vi "InitializeMotor.vi"(8 "error in":errorcluster) -> (0 "error out":errorcluster, 3 "Motor Ref":T1)   [LabVIEW 2016]
uses:
  <vilib>/myRIO/Instrument Drivers/Onboard IO/PWM/typedefs/PWM Configuration.ctl
  <vilib>/myRIO/Instrument Drivers/Onboard IO/PWM/PWM.lvlib
  <vilib>/myRIO/Common/Instrument Driver Framework/myRIO v1.0/PWM/typedefs/PWM Channels Enum.ctl
  <vilib>/myRIO/Common/Instrument Driver Framework/Utilities/typedefs/Generic FPGA Reference.ctl
  <vilib>/myRIO/Common/Instrument Driver Framework/Utilities/typedefs/myRIO v1.0 Reference.ctl
  <vilib>/myRIO/Common/Instrument Driver Framework/Utilities/typedefs/Hardware Version Enum.ctl
  <vilib>/myRIO/Common/Instrument Driver Framework/Utilities/typedefs/myRIO Generic Hardware Reference.ctl
  <vilib>/myRIO/Instrument Drivers/Onboard IO/PWM/typedefs/PWM Reference.ctl
  <vilib>/myRIO/Instrument Drivers/Onboard IO/PWM/vis/myRIO PWM Open.xnode
  <vilib>/myRIO/Common/Instrument Driver Framework/myRIO v1.0/PWM/vis/myRIO v1.1 Open PWM.vi
  <vilib>/userdefined/High Color/nirio_resource_hc.ctl
  <vilib>/myRIO/Common/Instrument Driver Framework/myRIO v1.0/DIO/typedefs/DIO Channels Enum.ctl
  <vilib>/myRIO/Common/Instrument Driver Framework/myRIO v1.0/DIO/typedefs/DIO Channels List.ctl
  <vilib>/myRIO/Instrument Drivers/Onboard IO/DIO/typedefs/DIO Reference.ctl
  <vilib>/myRIO/Instrument Drivers/Onboard IO/DIO/DIO.lvlib
  <vilib>/myRIO/Instrument Drivers/Onboard IO/DIO/vis/myRIO DIO Open.xnode
  <vilib>/myRIO/Common/Instrument Driver Framework/myRIO v1.0/DIO/vis/myRIO v1.1 Open DIO.vi
  <vilib>/myRIO/Common/Instrument Driver Framework/myRIO v1.0/Encoder/typedefs/Encoder Channels Enum.ctl
  <vilib>/myRIO/Instrument Drivers/Onboard IO/Encoder/typedefs/Encoder Reference.ctl
  <vilib>/myRIO/Instrument Drivers/Onboard IO/Encoder/Encoder.lvlib
  <vilib>/myRIO/Common/Instrument Driver Framework/myRIO v1.0/Encoder/typedefs/Encoder Signal Mode.ctl
  <vilib>/myRIO/Instrument Drivers/Onboard IO/Encoder/vis/myRIO Encoder Open.xnode
  <vilib>/myRIO/Common/Instrument Driver Framework/myRIO v1.0/Encoder/vis/myRIO v1.1 Open Encoder.vi
  <vilib>/myRIO/Common/Instrument Driver Framework/myRIO v1.0/Encoder/vis/myRIO v1.0 Configure Encoder.vi
  <vilib>/myRIO/Common/Instrument Driver Framework/myRIO v1.0/Encoder/typedefs/Encoder Configuration v1.0.ctl
  MotorObject.ctl
panel:
  in  "Motor Object":T1
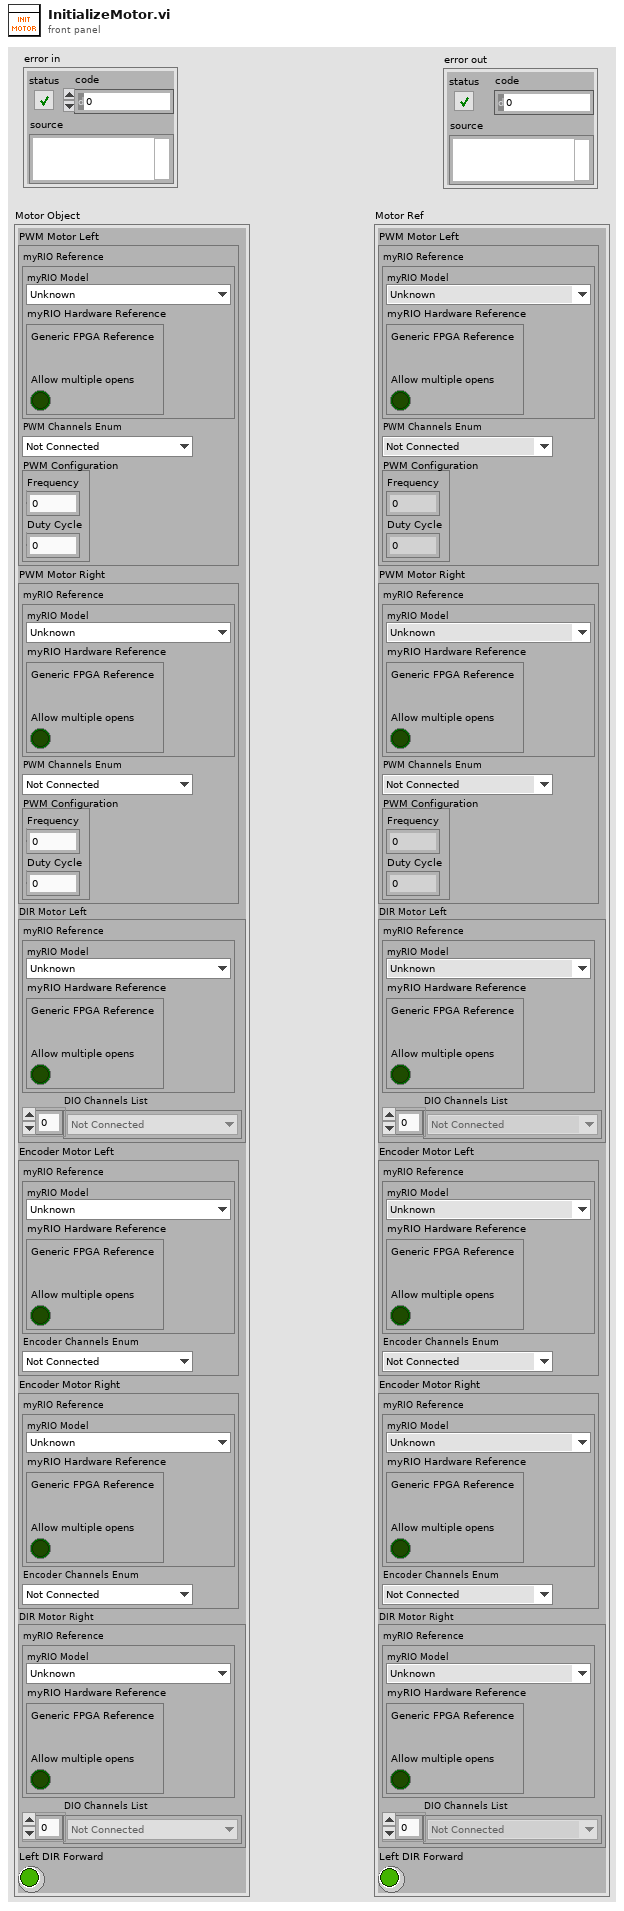
[diagram p1: front panel]
types:
  T1 = typedef "MotorObject.ctl" = cluster{"PWM Motor Left":T2, "PWM Motor Right":T2, "DIR Motor Left":T9, "Encoder Motor Left":T12, "Encoder Motor Right":T12, "DIR Motor Right":T9, "Left DIR Forward":bool}
  T2 = typedef "PWM.lvlib/PWM Reference.ctl" = cluster{"myRIO Reference":T3, "PWM Channels Enum":T7, "PWM Configuration":T8}
  T3 = typedef "myRIO Generic Hardware Reference.ctl" = cluster{"myRIO Model":T4, "myRIO Hardware Reference":T5}
  T4 = typedef "Hardware Version Enum.ctl" = enum16{"Unknown", "myRIO-1900", "myRIO-1950", "roboRIO", "NI ELVIS RIO CM"}
  T5 = typedef "myRIO v1.0 Reference.ctl" = cluster{"Generic FPGA Reference":T6, "Allow multiple opens":bool}
  T6 = typedef "Generic FPGA Reference.ctl" = refnum<k20>
  T7 = typedef "PWM Channels Enum.ctl" = enum16{"Not Connected", "C/PWM0", "C/PWM1", "A/PWM0", "A/PWM1", "A/PWM2", "B/PWM0", "B/PWM1", "B/PWM2", "PWM/PWM0", "PWM/PWM1", "PWM/PWM2", "PWM/PWM3", "PWM/PWM4", "PWM/PWM5", "PWM/PWM6", "PWM/PWM7", "PWM/PWM8", "PWM/PWM9"}
  T8 = typedef "PWM.lvlib/PWM Configuration.ctl" = cluster{"Frequency":dbl, "Duty Cycle":dbl}
  T9 = typedef "DIO.lvlib/DIO Reference.ctl" = cluster{"myRIO Reference":T3, "DIO Channels List":T10}
  T10 = typedef "DIO Channels List.ctl" = T11[]
  T11 = typedef "DIO Channels Enum.ctl" = enum16{"Not Connected", "C/DIO0", "C/DIO1", "C/DIO2", "C/DIO3", "C/DIO4", "C/DIO5", "C/DIO6", "C/DIO7", "A/DIO0", "A/DIO1", "A/DIO2", "A/DIO3", "A/DIO4", "A/DIO5", "A/DIO6", "A/DIO7", "A/DIO8", "A/DIO9", "A/DIO10", "A/DIO11", "A/DIO12", "A/DIO13", "A/DIO14", "A/DIO15", "B/DIO0", "B/DIO1", "B/DIO2", "B/DIO3", "B/DIO4", "B/DIO5", "B/DIO6", "B/DIO7", "B/DIO8", "B/DIO9", "B/DIO10", "B/DIO11", "B/DIO12", "B/DIO13", "B/DIO14", "B/DIO15", "LED0", "LED1", "LED2", "LED3", "Button0", "DIO/DIO0", "DIO/DIO1", "DIO/DIO2", "DIO/DIO3", "DIO/DIO4", "DIO/DIO5", "DIO/DIO6", "DIO/DIO7", "DIO/DIO8", "DIO/DIO9", "SPI/CS0", "SPI/CS1", "SPI/CS2", "SPI/CS3", "LED RADIO (Green)", "LED RADIO (Red)", "LED COMM (Green)", "LED COMM (Red)", "LED MODE (Green)", "LED MODE (Red)"}
  T12 = typedef "Encoder.lvlib/Encoder Reference.ctl" = cluster{"myRIO Reference":T3, "Encoder Channels Enum":T13}
  T13 = typedef "Encoder Channels Enum.ctl" = enum16{"Not Connected", "C/ENC0", "C/ENC1", "A/ENC", "B/ENC", "DIO/ENC0", "DIO/ENC1", "DIO/ENC2", "DIO/ENC3", "DIO/ENC4"}
  T14 = typedef "nirio_resource_hc.ctl" = tag
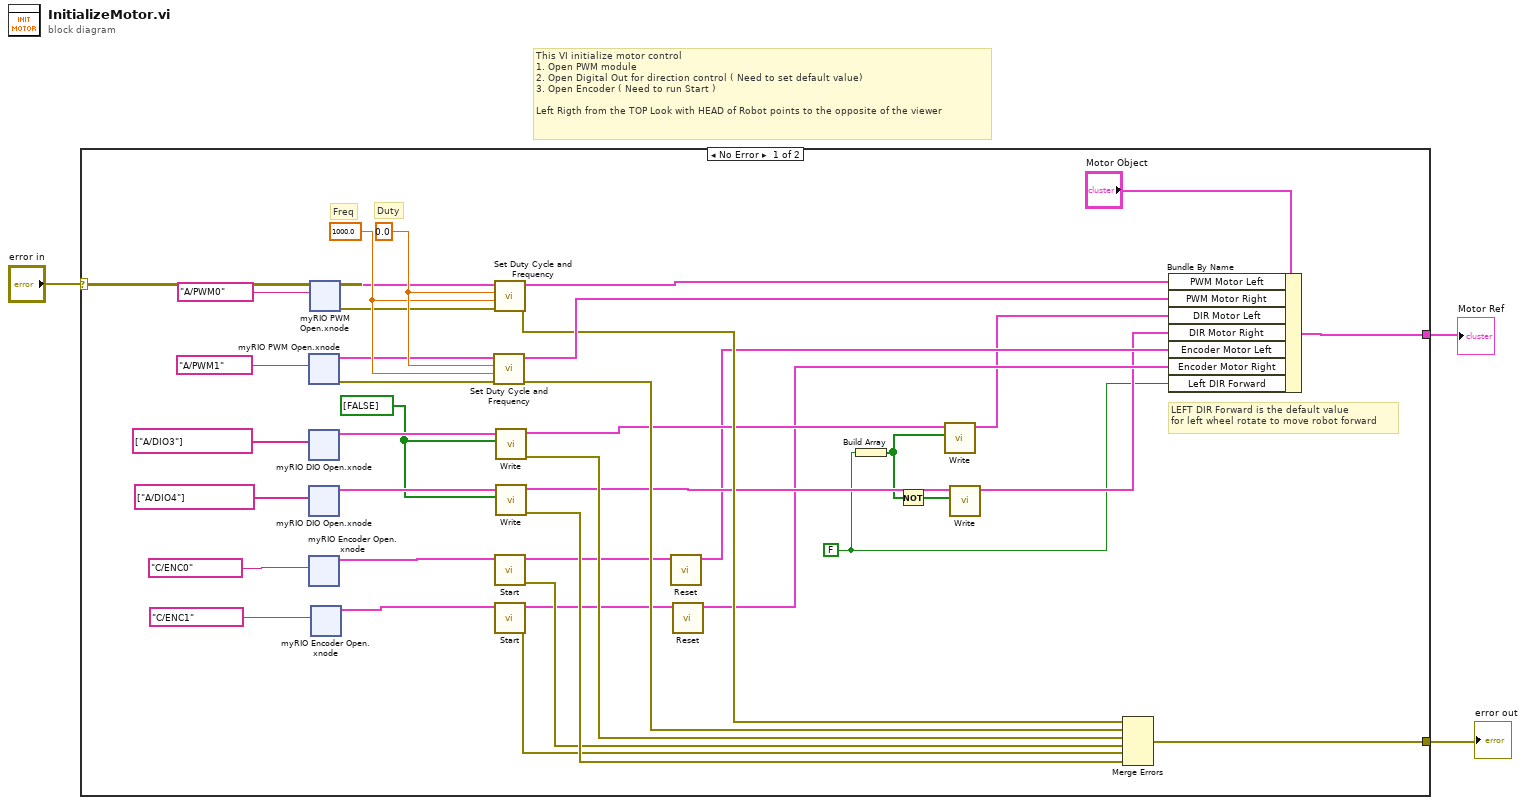
[diagram p0: block diagram]
diagram:
  # "This VI initialize motor control\n1. Open PWM module\n2. Open Digital Out for direction control ( Need to set default value)\n3. Open Encoder ( Need to run Start )\n\nLeft Rigth from the TOP Look with HEAD of Robot points to the opposite of the viewer"
  n1 = case shown="No Error" "error in" {
    selector: "error in" -> [_ w149]
    tunnel: [w20 _] -> w2
    tunnel: [w18 w149] -> w1
    frame No Error {
      w6 = FALSE ("Left DIR Forward")
      w17 = bool[] [FALSE] ("Values")
      w30 = 0.0 ("Duty Cycle")
      w29 = 1000.0 ("Frequency [Hz]")
      # "LEFT DIR Forward is the default value\nfor left wheel rotate to move robot forward"
      # "Duty"
      # "Freq"
      n2 = xnode "myRIO PWM Open.xnode"("Channel Name"=tag "A/PWM1") -> ("error out"=w28:errorcluster, "PWM Ref Out"=w24:T2)  [unwired: 2 in]
      n3 = xnode "myRIO DIO Open.xnode"("Channel Names"=tag[] ["A/DIO3"]) -> ("DIO Ref Out"=w33:T9)  [unwired: 2 in, 1 out]
      n4 = xnode "myRIO DIO Open.xnode"("Channel Names"=tag[] ["A/DIO4"]) -> ("DIO Ref Out"=w37:T9)  [unwired: 2 in, 1 out]
      n5 = xnode "myRIO Encoder Open.xnode"("Channel Name"=tag "C/ENC0") -> ("Encoder Ref Out"=w41:T12)  [unwired: 4 in, 1 out]
      n6 = xnode "myRIO PWM Open.xnode"("Channel Name"=tag "A/PWM0") -> ("error out"=w27:errorcluster, "PWM Ref Out"=w21:T2)  [unwired: 2 in]
      n7 = xnode "myRIO Encoder Open.xnode"("Channel Name"=tag "C/ENC1") -> ("Encoder Ref Out"=w42:T12)  [unwired: 4 in, 1 out]
      n8 = call <vilib>:"Set Duty Cycle and Frequency.vi"("error in (no error)"=w28, "Frequency [Hz]"=w29, "Duty Cycle"=w30, "PWM Ref In"=w24) -> ("error out"=w32:errorcluster, "PWM Ref Out"=w36:T2)  [unwired: 5 in]
      n9 = call <vilib>:"Set Duty Cycle and Frequency.vi"("error in (no error)"=w27, "Frequency [Hz]"=w29, "Duty Cycle"=w30, "PWM Ref In"=w21) -> ("error out"=w31:errorcluster, "PWM Ref Out"=w35:T2)  [unwired: 5 in]
      n10 = call <vilib>:"Start.vi"("Encoder Ref In"=w41) -> ("error out"=w16:errorcluster, "Encoder Ref Out"=w14:T12)  [unwired: 9 in]
      n11 = call <vilib>:"Start.vi"("Encoder Ref In"=w42) -> ("error out"=w15:errorcluster, "Encoder Ref Out"=w13:T12)  [unwired: 9 in]
      n12 = call <vilib>:"Write.vi"("Values"=w17, "DIO Ref In"=w33) -> ("error out"=w34:errorcluster, "DIO Ref Out"=w12:T9)  [unwired: 7 in]
      n13 = call <vilib>:"Write.vi"("Values"=w17, "DIO Ref In"=w37) -> ("error out"=w38:errorcluster, "DIO Ref Out"=w11:T9)  [unwired: 7 in]
      n14 = call <vilib>:"Reset.vi"("Encoder Ref In"=w14) -> ("Encoder Ref Out"=w10:T12)  [unwired: 9 in, 1 out]
      n15 = call <vilib>:"Reset.vi"("Encoder Ref In"=w13) -> ("Encoder Ref Out"=w9:T12)  [unwired: 9 in, 1 out]
      n16 = Build Array(w6) -> (w4:bool[])
      n17 = Not(x=w4) -> (.not. x?=w5:bool[])
      n18 = call <vilib>:"Write.vi"("Values"=w4, "DIO Ref In"=w12) -> ("DIO Ref Out"=w7:T9)  [unwired: 7 in, 1 out]
      n19 = call <vilib>:"Write.vi"("Values"=w5, "DIO Ref In"=w11) -> ("DIO Ref Out"=w8:T9)  [unwired: 7 in, 1 out]
      n20 = Merge Errors(w31, w32, w34, w16, w15, w38) -> (w18:errorcluster)
      n21 = Bundle By Name(cluster="Motor Object", "PWM Motor Left"=w35, "PWM Motor Right"=w36, "DIR Motor Left"=w7, "DIR Motor Right"=w8, "Encoder Motor Left"=w10, "Encoder Motor Right"=w9, "Left DIR Forward"=w6) -> (w20:T1)
    }
    frame Error {
    }
  }
  "Motor Ref" <- w2
  "error out" <- w1
